vi "DC Step.vi"(8 "error in (no error)":errorcluster, 10 "DC Offset":dbl, 11 "PXIe5413 in":refnum<class "PXIe5413.lvclass">) -> (0 "error out":errorcluster, 3 "PXIe5413 out":refnum<class "PXIe5413.lvclass">)   [LabVIEW 2018, in "PXIe5413.lvlib" / "PXIe5413.lvclass"]
uses:
  PXIe5413.lvclass
  PXIe5413.lvclass/PXIe5413.ctl
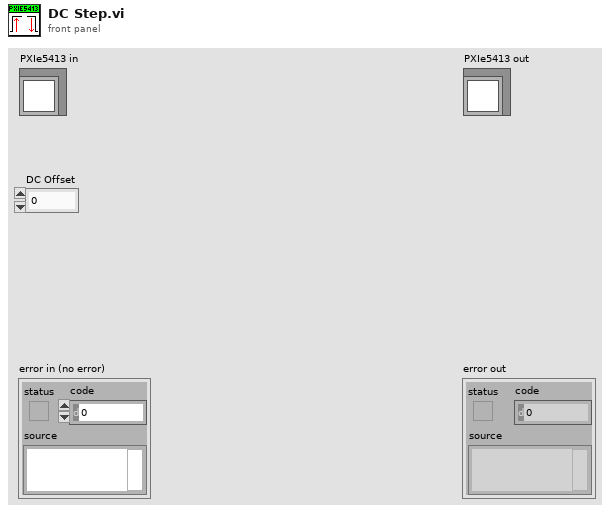
[diagram p1: front panel]
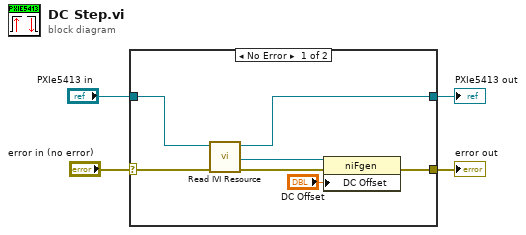
[diagram p0: block diagram]
diagram:
  n1 = case shown="No Error" "error in (no error)" {
    selector: "error in (no error)" -> [w10 w13]
    tunnel: [w5 w13] -> w3
    tunnel: [w6 w12] -> w2
    tunnel: "PXIe5413 in" -> [w11 w12]
    frame No Error {
      n2 = call "Read IVI Resource.vi"("error in (no error)"=w10, "PXIe5413 in"=w11) -> ("error out"=w9:errorcluster, "IVI Resource"=w8:refnum<k15>, "PXIe5413 out"=w6:refnum<class "PXIe5413.lvclass">)  [unwired: 7 in]
      n3 = property class="niFgen"(reference=w8, error in=w9, "DC Offset"="DC Offset") -> (error out=w5:errorcluster)  [unwired: 1 out]
    }
    frame Error {
    }
  }
  "error out" <- w3
  "PXIe5413 out" <- w2
